vi "AverageFFT.vi"() -> ()   [LabVIEW 2015]
uses:
  <vilib>/express/express analysis/Spectral/Block/exnSpectralBlock spectral measurements RMS poly.vi
  <vilib>/express/express analysis/Spectral/Block/exnSpectralBlock spectral measurements RMS DDT.vi
  <vilib>/express/express analysis/Spectral/XNode/ExpressSpectralMeasurementsBlockNode.xnode
panel:
  out "error out":errorcluster
  in  "error in":errorcluster
  out "FFT":dynamicdata(graph)
  out "?":dbl[](graph)
  in  "?":bool
  in  "Time (s)":dbl
  in  "Rate":dbl
  in  "Averages":dbl
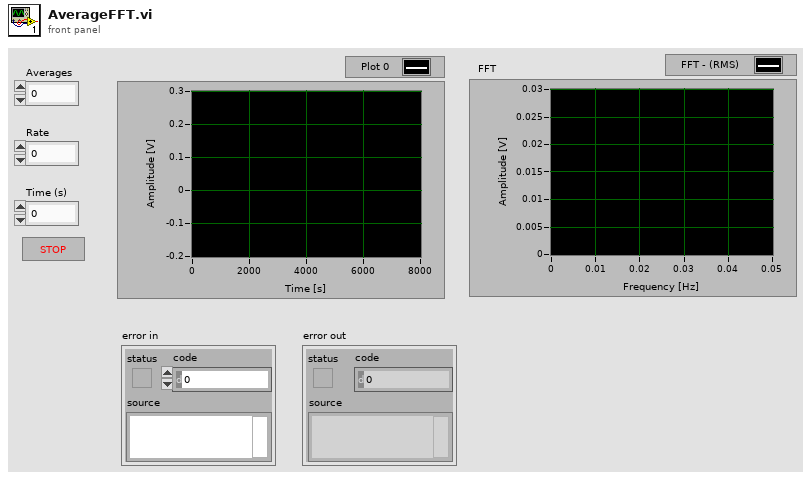
[diagram p1: front panel]
types:
  T1 = cluster{"averaging mode":u16, "weighting mode":u16, "number of averages":u32}
  T2 = cluster{"dB On (F)":bool, "unwrap phase (F)":bool, "convert to degree (F)":bool}
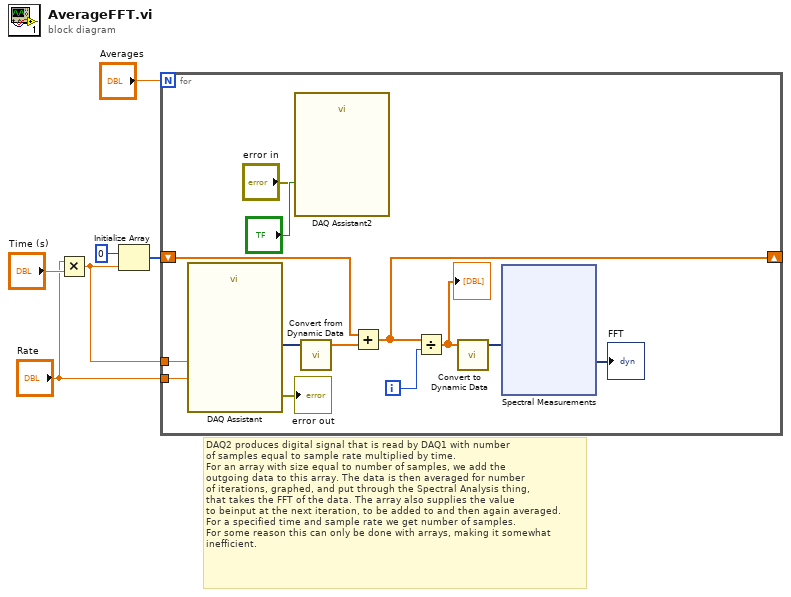
[diagram p0: block diagram]
diagram:
  # "DAQ2 produces digital signal that is read by DAQ1 with number\nof samples equal to sample rate multiplied by time.\nFor an array with size equal to number of samples, we add the\noutgoing data to this array. The data is then averaged for number\nof iterations, graphed, and put through the Spectral Analysis thing,\nthat takes the FFT of the data. The array also supplies the value\nto beinput at the next iteration, to be added to and then again averaged.\nFor a specified time and sample rate we get number of samples.\nFor some reason this can only be done with arrays, making it somewhat\ninefficient."
  n1 = Multiply(x="Rate", y="Time (s)") -> (x*y=w2:dbl)
  n2 = Initialize Array(0, w2) -> (w1:i32[])
  n3 = for {
    N: "Averages" -> [_]
    shift-right: [w7] -> _
    shift-left: w1 -> [w19]
    tunnel: w2 -> [w14]
    tunnel: "Rate" -> [w15]
    i -> [w18]
    n4 = call "DAQ Assistant"("rate"=w15, "number of samples"=w14) -> ("data"=w11:dynamicdata, "error out"=→"error out":errorcluster)  [unwired: 15 in, 1 out]
    n5 = call "DAQ Assistant2"("error in"="error in", "stop (T)"="?") -> ()  [unwired: 16 in, 2 out]
    n6 = call "Convert from Dynamic Data"("Dynamic Data Type"=w11) -> ("Array"=w16:dbl[])  [unwired: 3 in]
    n7 = Add(x=w19, y=w16) -> (x+y=w7:dbl[])
    n8 = Divide(x=w7, y=w18) -> (x/y=w9:dbl[])
    "?" <- w9
    n9 = call "Convert to Dynamic Data"("Array"=w9) -> ("Dynamic Data Type"=w8:dynamicdata)  [unwired: 3 in]
    n10 = xnode "Spectral Measurements"("Signals"=w8) -> ("FFT - (RMS)"=→"FFT":dynamicdata)  [unwired: 1 in, 2 out]
  }
